vi "GetVersionChain.vi"(8 "error in (no error)":errorcluster, 11 "reference in":refnum<class "Component_Template.lvclass">) -> (0 "error out":errorcluster, 2 "Version Chain":T1(array[cluster]), 3 "reference in":refnum<class "Component_Template.lvclass">)   [LabVIEW 2022 SP3, in "Component_Template.lvlib" / "Component_Template.lvclass"]
uses:
  Component_Template.lvclass
  Components/ViPER.lvlibp/ViPER.lvclass
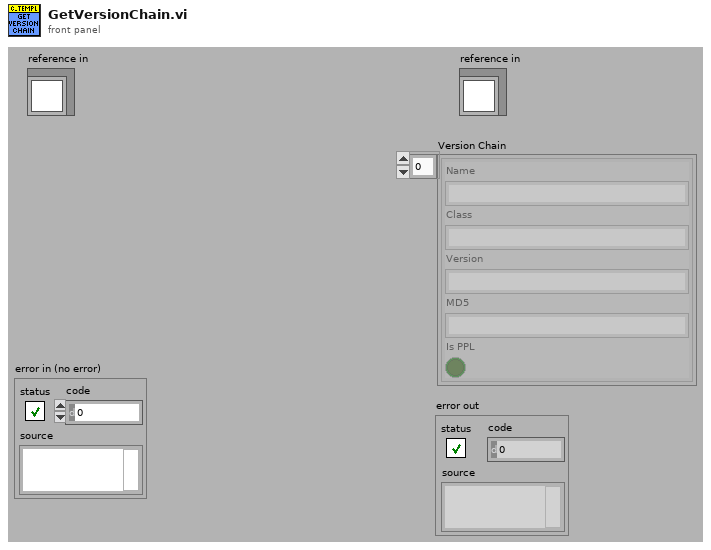
[diagram p1: front panel]
types:
  T1 = cluster{"Name":string, "Class":string, "Version":string, "MD5":string, "Is PPL":bool}[]
  T2 = cluster{"Name":string, "Class":string, "Version":string, "MD5":string, "Is PPL":bool}
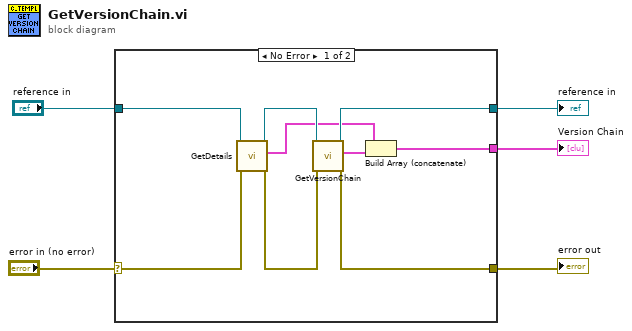
[diagram p0: block diagram]
diagram:
  n1 = case shown="No Error" "error in (no error)" {
    selector: "error in (no error)" -> [w10 w16]
    tunnel: [w13 w16] -> w4
    tunnel: [w14 w15] -> w2
    tunnel: "reference in" -> [w12 w15]
    tunnel: [w6 _] -> w1
    frame No Error {
      n2 = call-dynamic "GetDetails.vi"("error in (no error)"=w10, "reference in"=w12) -> ("error out"=w9:errorcluster, "Details"=w7:T2, "reference out"=w11:refnum<class "Component_Template.lvclass">)  [unwired: 7 in]
      n3 = call-parent "GetVersionChain.vi"("error in (no error)"=w9, "reference in"=w11) -> ("error out"=w13:errorcluster, "Version Chain"=w8:T1, "reference out"=w14:refnum<class "Component_Template.lvclass">)  [unwired: 7 in]
      n4 = Build Array (concatenate)(w7, w8) -> (w6:T1)
    }
    frame Error {
    }
  }
  "error out" <- w4
  "reference in" <- w2
  "Version Chain" <- w1
